vi "AuMT8852B Tester Pin Code.vi"(5 "Pin Code (0000)":string, 7 "Set/Get (Set) 4":enum16{"Set", "Get"}(ring), 8 "error in (no error)":errorcluster, 10 "Length (4)":i32, 11 "VISA session":refnum<visa-resource-name>) -> (0 "error out":errorcluster, 2 "error code":i32, 3 "VISA session out":refnum<visa-resource-name>, 4 "Pin Code out":string)   [LabVIEW 2017]
doc: "Anritsu MT8852B Bluetooth Tester\n\nControls the pin code used for authentication.\n\nINPUTS\nSet/Get - whether the value is being sent to or retrieved from the instrument.\nPin Code - the code to be sent to the instrument.\nLength - the number of characters used in the code.\n\nOUTPUTS\nPin Code out - the current pin code stored within the instrument."
uses:
  <instrlib>/aumt8852B/General/Utilities/MT8850 Attribute ID.ctl
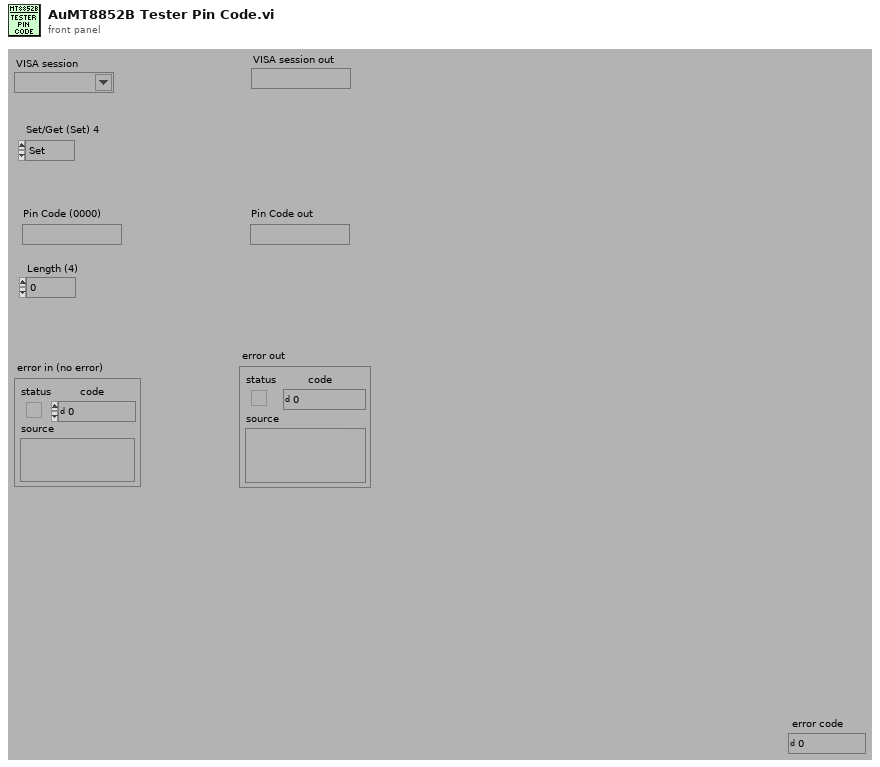
[diagram p1: front panel]
types:
  T1 = typedef "MT8850 Attribute ID.ctl" = enum16{"Operation mode", "Selected script", "EUT address source", "EUT Address", "EUT HCI RS232 Baud Rate", "Tester GPIB Address", "Tester RS232 Baud Rate", "Tester Bluetooth Address", "Tester Contrast", "Tester Key Click On", "Tester Modulation Index", "Tester Poll-Null Mode", "Tester Power Range", "Tester RS232 Mode", "Beep on Illegal Entry", "Display User Text", "User Text", "Calibration TX Modulation DAC", "Calibration RX Channel", "Calibration TX Channel", "Calibration TX Power", "Calibration Use TX Table", "Inquiry Request User-friendly Name", "Inquiry Number of Responses", "Inquiry Timeout", "Script Frequency Display", "Script Loop Count", "Script Loop Continuously", "Script Loop Stop on Fail", "Link timeout", "Page timeout", "Filter bandwidth", "SCO air code", "SCO bit position", "SCO input code", "SCO input data", "SCO input sample size", "SCO loopback mode", "SCO packet type", "SCO tone generator", "Tester page scan repetition mode", "Tester follow test mode", "Tester authentication state", "Tester authentication pin code", "Tester authentication pin length"}
  T2 = typedef "Attribute Status.ctl" = enum16{"No I/O needed", "I/O needed"}
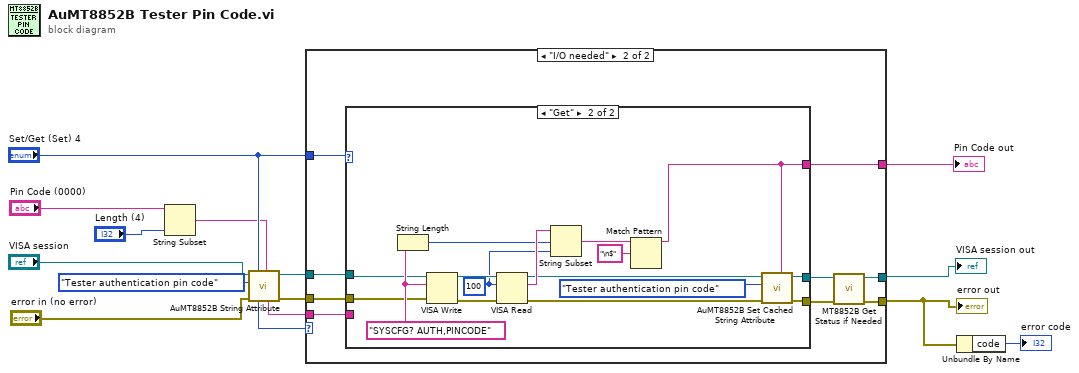
[diagram p0: block diagram]
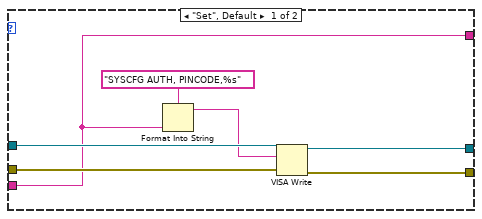
[diagram p3: hidden frame]
diagram:
  n1 = String Subset(string="Pin Code (0000)", length (rest)="Length (4)") -> (substring=w2:string)  [unwired: 1 in]
  n2 = call <instrlib>:"AuMT8852B String Attribute.vi"("Value (\"\")"=w2, "Set/Get (Set)"="Set/Get (Set) 4", "error in (no error)"="error in (no error)", "Attribute ID"=MT8850_Attribute_ID."Tester authentication pin code", "VISA session"="VISA session") -> ("error out"=w6:errorcluster, "VISA session out"=w7:refnum<visa-resource-name>, "Value out"=w5:string, "Status"=w12:T2)  [unwired: 3 in]
  n3 = case shown="\"I/O needed\"" w12 {
    tunnel: [w16 w26] -> w15
    tunnel: [w17 w27] -> w13
    tunnel: "Set/Get (Set) 4" -> [_ w23]
    tunnel: w5 -> [w18 w20]
    tunnel: w6 -> [w17 w22]
    tunnel: w7 -> [w16 w21]
    tunnel: [w18 w19] -> w4
    frame "No I/O needed", Default {
    }
    frame "I/O needed" {
      n4 = case shown="\"Get\"" w23 {
        tunnel: [w29 w40] -> w24
        tunnel: [w30 w41] -> w25
        tunnel: w22 -> [w34 w44]
        tunnel: w21 -> [w33 w43]
        tunnel: w20 -> [w28 _]
        tunnel: [w28 w35] -> w19
        frame "Set", Default {
          n5 = Format Into String(format string="SYSCFG AUTH, PINCODE,%s", w28) -> (resulting string=w31:string)  [unwired: 2 in, 1 out]
          n6 = VISA Write(VISA resource name=w33, write buffer=w31, error in (no error)=w34) -> (VISA resource name out=w29:refnum<visa-resource-name>, error out=w30:errorcluster)  [unwired: 1 out]
        }
        frame "Get" {
          w45 = u32 100 ("byte count (0)")
          w47 = "SYSCFG? AUTH,PINCODE" ("write buffer (\"\")")
          n7 = String Length(string=w47) -> (length=w46:i32)
          n8 = VISA Write(VISA resource name=w43, write buffer=w47, error in (no error)=w44) -> (VISA resource name out=w50:refnum<visa-resource-name>, error out=w49:errorcluster)  [unwired: 1 out]
          n9 = VISA Read(VISA resource name=w50, byte count=w45, error in (no error)=w49) -> (VISA resource name out=w39:refnum<visa-resource-name>, read buffer=w48:string, error out=w42:errorcluster)  [unwired: 1 out]
          n10 = String Subset(string=w48, offset (0)=w46, length (rest)=w45) -> (substring=w36:string)
          n11 = Match Pattern(string=w36, regular expression="\n$") -> (before substring=w35:string)  [unwired: 1 in, 3 out]
          n12 = call <instrlib>:"AuMT8852B Set Cached String Attribute.vi"("Value (\"\")"=w35, "error in (no error)"=w42, "Attribute ID"=MT8850_Attribute_ID."Tester authentication pin code", "VISA session"=w39) -> ("error out"=w41:errorcluster, "VISA session out"=w40:refnum<visa-resource-name>)  [unwired: 6 in]
        }
      }
      n13 = call <instrlib>:"MT8852B Get Status if Needed.vi"("error in (no error)"=w25, "VISA session"=w24) -> ("error out"=w27:errorcluster, "VISA session out"=w26:refnum<visa-resource-name>)  [unwired: 8 in]
    }
  }
  "VISA session out" <- w15
  "error out" <- w13
  "Pin Code out" <- w4
  n14 = Unbundle By Name(w13) -> ("code"=→"error code":i32)
